vi "ESP300currentposition2.vi"(4 "error in (no error)":errorcluster, 6 "ESP300Axis":string, 7 "ESP300Address":string) -> (0 "error out":errorcluster, 3 "Current Position":dbl)   [LabVIEW 2010]
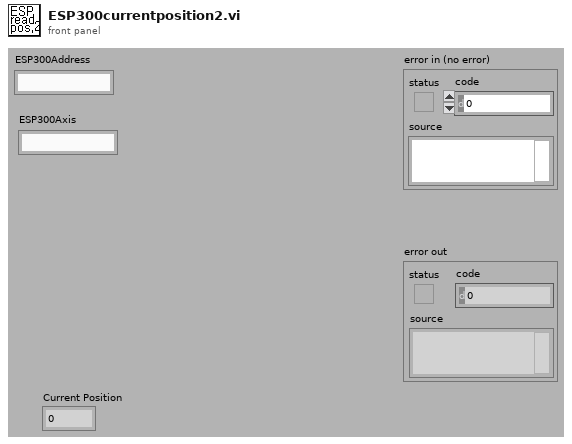
[diagram p1: front panel]
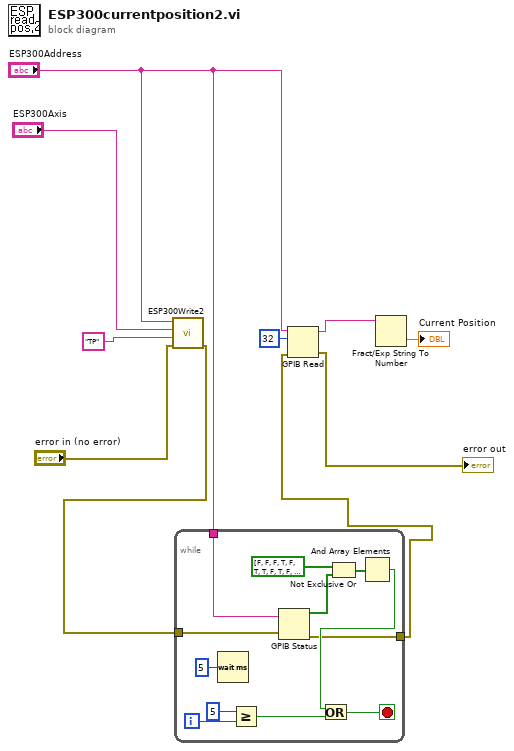
[diagram p0: block diagram]
diagram:
  n1 = call "ESP300Write2.vi"("error in (no error)"="error in (no error)", "Command"="TP", "ESP300 Channel"="ESP300Axis", "ESP300 Address"="ESP300Address") -> ("error out"=w3:errorcluster)  [unwired: 3 in]
  n2 = while {
    tunnel: w3 -> [w22]
    tunnel: [w12] -> w2
    tunnel: "ESP300Address" -> [w11]
    i -> [w21]
    stop <- w18 stop-if-true
    n3 = Wait (ms)(milliseconds to wait=u32 5) -> ()  [unwired: 1 out]
    n4 = Greater Or Equal?(x=5, y=w21) -> (x >= y?=w19:bool)
    n5 = GPIB Status(0:w11, 1:w22) -> (2:w16:bool[], 5:w12:errorcluster)  [unwired: 2 out]
    n6 = Not Exclusive Or(1:w16, 2:bool[] [FALSE, FALSE, FALSE, TRUE, FALSE, TRUE, TRUE, FALSE, TRUE, FALSE, FALSE, FALSE, FALSE, FALSE, FALSE, FALSE] ("status 2")) -> (0:w15:bool[])
    n7 = And Array Elements(Boolean array=w15) -> (logical AND=w14:bool)
    n8 = Or(x=w14, y=w19) -> (x .or. y?=w18:bool)
  }
  n9 = GPIB Read(0:"ESP300Address", 1:32 ("byte count"), 3:w2) -> (5:w8:string, 7:→"error out":errorcluster)  [unwired: 2 in, 1 out]
  n10 = Fract/Exp String To Number(string=w8) -> (number=→"Current Position":dbl)  [unwired: 3 in, 1 out]
